vi "LTVUnicycleCtrl_Calculate_TrajState.vi"(9 "TRAJ_STATE":T1={"TimeSeconds"=0.0, "Velocity"=0.0, "Acceleration"=0.0, "POSE"={"TRANSLATION"={"X"=0.0, "Y"=0.0}, "ROTATION"={"VALUE"=0.0, "COS"=1.0, "SIN"=0.0}}, "Curvature"=0.0} {"POSE"."ROTATION"."SIN" format="%13.4f"; "POSE"."ROTATION"."COS" format="%13.4f"; "POSE"."ROTATION"."VALUE" format="%13.4f"; "POSE"."TRANSLATION"."Y" format="%14.3f"; "POSE"."TRANSLATION"."X" format="%14.3f"}, 10 "CurrentPose":T2={"TRANSLATION"={"X"=0.0, "Y"=0.0}, "ROTATION"={"VALUE"=0.0, "COS"=1.0, "SIN"=0.0}} {"ROTATION"."SIN" format="%13.4f"; "ROTATION"."COS" format="%13.4f"; "ROTATION"."VALUE" format="%13.4f"; "TRANSLATION"."Y" format="%14.3f"; "TRANSLATION"."X" format="%14.3f"}, 11 "in LTV_UNICYCLE_CONTROLLER":T6={"m_A"=[], "m_B"=[], "m_Q"=[], "m_R"=[], "States"=0, "Inputs"=0, "PoseError"={"TRANSLATION"={"X"=0.0, "Y"=0.0}, "ROTATION"={"VALUE"=0.0, "COS"=1.0, "SIN"=0.0}}, "PoseTolerance"={"TRANSLATION"={"X"=0.0, "Y"=0.0}, "ROTATION"={"VALUE"=0.0, "COS"=1.0, "SIN"=0.0}}, "Dt"=0.02, "Enabled"=FALSE, "savedLQR_K"={"Table Xs"=[], "Table Ys"=[], "MinX"=0.0, "MaxX"=0.0, "ItemCount"=0, "Rows"=0, "Columns"=0}} {"PoseTolerance"."ROTATION"."SIN" format="%13.4f"; "PoseTolerance"."ROTATION"."COS" format="%13.4f"; "PoseTolerance"."ROTATION"."VALUE" format="%13.4f"; "PoseTolerance"."TRANSLATION"."Y" format="%14.3f"; "PoseTolerance"."TRANSLATION"."X" format="%14.3f"; "PoseError"."ROTATION"."SIN" format="%13.4f"; "PoseError"."ROTATION"."COS" format="%13.4f"; "PoseError"."ROTATION"."VALUE" format="%13.4f"; "PoseError"."TRANSLATION"."Y" format="%14.3f"; "PoseError"."TRANSLATION"."X" format="%14.3f"}) -> (0 "Error":bool, 2 "ChassisSpeeds":T5 {"vOmega" format="%10.3f"; "vY" format="%10.3f"; "vX" format="%10.3f"}, 3 "out LTV_UNICYCLE_CONTROLLER":T6={"m_A"=[], "m_B"=[], "m_Q"=[], "m_R"=[], "States"=0, "Inputs"=0, "PoseError"={"TRANSLATION"={"X"=0.0, "Y"=0.0}, "ROTATION"={"VALUE"=0.0, "COS"=1.0, "SIN"=0.0}}, "PoseTolerance"={"TRANSLATION"={"X"=0.0, "Y"=0.0}, "ROTATION"={"VALUE"=0.0, "COS"=1.0, "SIN"=0.0}}, "Dt"=0.02, "Enabled"=FALSE, "savedLQR_K"={"Table Xs"=[], "Table Ys"=[], "MinX"=0.0, "MaxX"=0.0, "ItemCount"=0, "Rows"=0, "Columns"=0}} {"PoseTolerance"."ROTATION"."SIN" format="%13.4f"; "PoseTolerance"."ROTATION"."COS" format="%13.4f"; "PoseTolerance"."ROTATION"."VALUE" format="%13.4f"; "PoseTolerance"."TRANSLATION"."Y" format="%14.3f"; "PoseTolerance"."TRANSLATION"."X" format="%14.3f"; "PoseError"."ROTATION"."SIN" format="%13.4f"; "PoseError"."ROTATION"."COS" format="%13.4f"; "PoseError"."ROTATION"."VALUE" format="%13.4f"; "PoseError"."TRANSLATION"."Y" format="%14.3f"; "PoseError"."TRANSLATION"."X" format="%14.3f"})   [LabVIEW 2019, in "Trajectory_Library.lvlib"]
doc: "Create implicit model follower\n\nInputs:\n - A < states, states > -- Continuous system matrix of the plant being controlled.\n - B < states, inputs > -- Continuous input matrix of the plant being controlled.\n - A_Ref < states, states > -- Continuous system matrix whose dymanics should be followed.\n - B_Ref < states, inputs > -- Continuous input matrix x whose dymanics should be followed.\n\nOutputs:\n - Error -- If TRUE, an error occured."
uses:
  Trajectory_Library.lvlib
  TypeDef/LTV_UNICYCLE_CONTROLLER.ctl
  <vilib>/Analysis/Matrix/Datatypes/RealMatrix.ctl
  TypeDef/POSE2D.ctl
  TypeDef/TRANSLATION2D.ctl
  TypeDef/ROTATION2D.ctl
  TypeDef/FUNCTION_GENERATOR_MATRIX.ctl
  TypeDef/CHASSIS_SPEEDS.ctl
  TypeDef/TRAJ_STATE.ctl
  <vilib>/Analysis/Matrix/NI_Matrix.lvlib
panel:
  # "<States,States>"
  # "<States,Inputs>"
  # "<States, States>"
  # "<Inputs, Inputs>"
  # "<States,States>"
  # "<States,Inputs>"
  # "<States, States>"
  # "<Inputs, Inputs>"
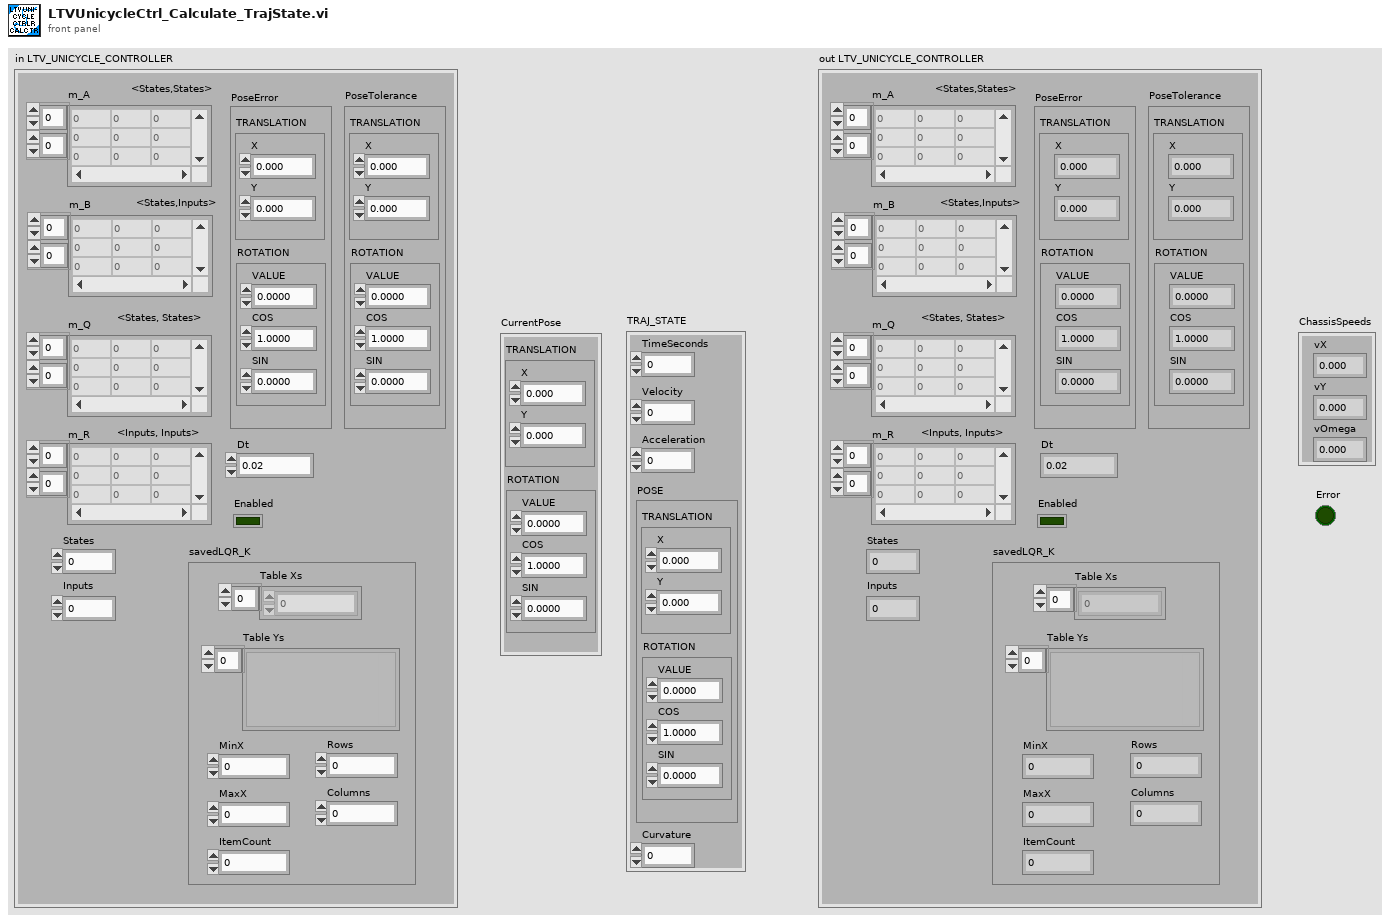
[diagram p1: front panel]
types:
  T1 = typedef "Trajectory_Library.lvlib/TRAJ_STATE.ctl" = cluster{"TimeSeconds":dbl, "Velocity":dbl, "Acceleration":dbl, "POSE":T2, "Curvature":dbl}
  T2 = typedef "Trajectory_Library.lvlib/POSE2D.ctl" = cluster{"TRANSLATION":T3, "ROTATION":T4}
  T3 = typedef "Trajectory_Library.lvlib/TRANSLATION2D.ctl" = cluster{"X":dbl, "Y":dbl}
  T4 = typedef "Trajectory_Library.lvlib/ROTATION2D.ctl" = cluster{"VALUE":dbl, "COS":dbl, "SIN":dbl}
  T5 = typedef "Trajectory_Library.lvlib/CHASSIS_SPEEDS.ctl" = cluster{"vX":dbl, "vY":dbl, "vOmega":dbl}
  T6 = typedef "Trajectory_Library.lvlib/LTV_UNICYCLE_CONTROLLER.ctl" = cluster{"m_A":T7, "m_B":T7, "m_Q":T7, "m_R":T7, "States":i32, "Inputs":i32, "PoseError":T2, "PoseTolerance":T2, "Dt":dbl, "Enabled":bool, "savedLQR_K":T8}
  T7 = typedef "NI_Matrix.lvlib/RealMatrix.ctl" = dbl[][]
  T8 = typedef "Trajectory_Library.lvlib/FUNCTION_GENERATOR_MATRIX.ctl" = cluster{"Table Xs":dbl[], "Table Ys":variant[], "MinX":dbl, "MaxX":dbl, "ItemCount":i32, "Rows":i32, "Columns":i32}
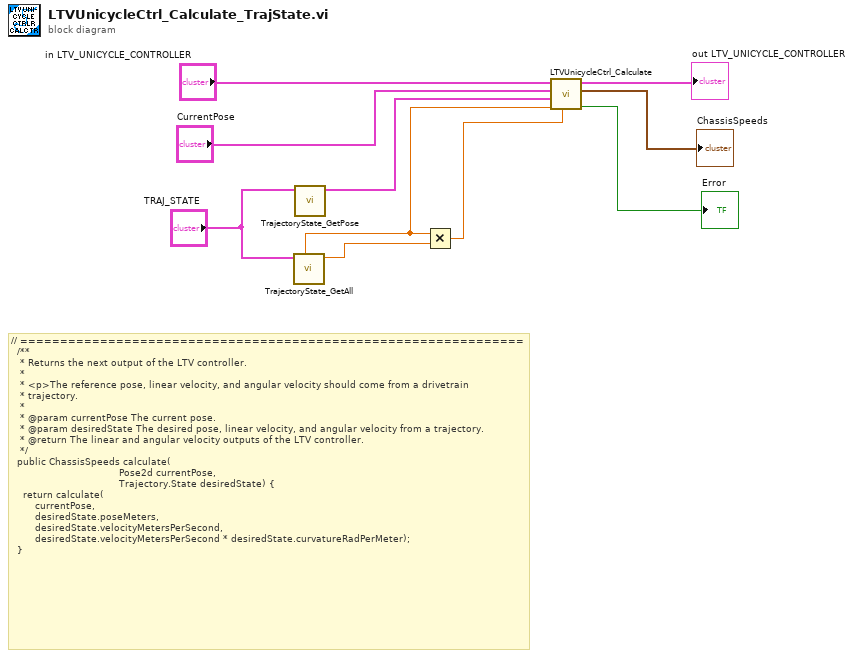
[diagram p0: block diagram]
diagram:
  # "// ===============================================================\n  /**\n   * Returns the next output of the LTV controller.\n   *\n   * <p>The reference pose, linear velocity, and angular velocity should come from a drivetrain\n   * trajectory.\n   *\n   * @param currentPose The current pose.\n   * @param desiredState The desired pose, linear velocity, and angular velocity from a trajectory.\n   * @return The linear and angular velocity outputs of the LTV controller.\n   */\n  public ChassisSpeeds calculate(\n                                    Pose2d currentPose, \n                                    Trajectory.State desiredState) {\n    return calculate(\n        currentPose,\n        desiredState.poseMeters,\n        desiredState.velocityMetersPerSecond,\n        desiredState.velocityMetersPerSecond * desiredState.curvatureRadPerMeter);\n  }"
  n1 = call "TrajectoryState_GetAll.vi"("TRAJ_STATE"="TRAJ_STATE") -> ("Curvature"=w2:dbl, "Velocity"=w3:dbl)  [unwired: 4 in, 5 out]
  n2 = call "TrajectoryState_GetPose.vi"("TRAJ_STATE"="TRAJ_STATE") -> ("TrajStatePose"=w5:T2)  [unwired: 10 in]
  n3 = Multiply(x=w3, y=w2) -> (x*y=w1:dbl)
  n4 = call "LTVUnicycleCtrl_Calculate.vi"("RefAngularVelocity"=w1, "RefLinearVelocity"=w3, "RefPose"=w5, "CurrentPose"="CurrentPose", "in LTV_UNICYCLE_CONTROLLER"="in LTV_UNICYCLE_CONTROLLER") -> ("Error"=→"Error":bool, "ChassisSpeeds"=→"ChassisSpeeds":T5, "out LTV_UNICYCLE_CONTROLLER"=→"out LTV_UNICYCLE_CONTROLLER":T6)  [unwired: 4 in]
